vi "Link Read Parameters.vi"(7 "Parameter R Table in":refnum<class "Registry.lvclass">, 8 "error in (no error)":errorcluster, 11 "Major Frame in":refnum<class "Major Frame.lvclass">) -> (0 "error out":errorcluster, 5 "Parameter R Table out":refnum<class "Registry.lvclass">)   [LabVIEW 2020, in "BCI-1553 API.lvlib" / "Major Frame.lvclass"]
doc: "Links read-only transmit parameters to the Read Table."
uses:
  Major Frame.lvclass
  Dependencies/Registry/Registry.lvclass
  Major Frame.lvclass/Major Frame.ctl
  Dependencies/Registry/Registry.lvclass/Registry.ctl
  Message/Message.lvclass
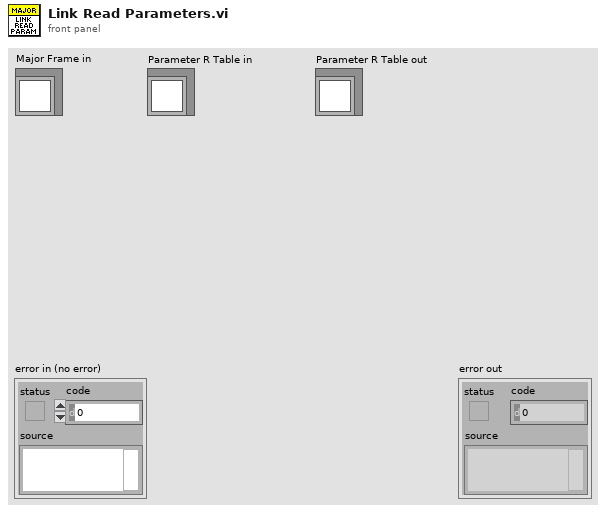
[diagram p1: front panel]
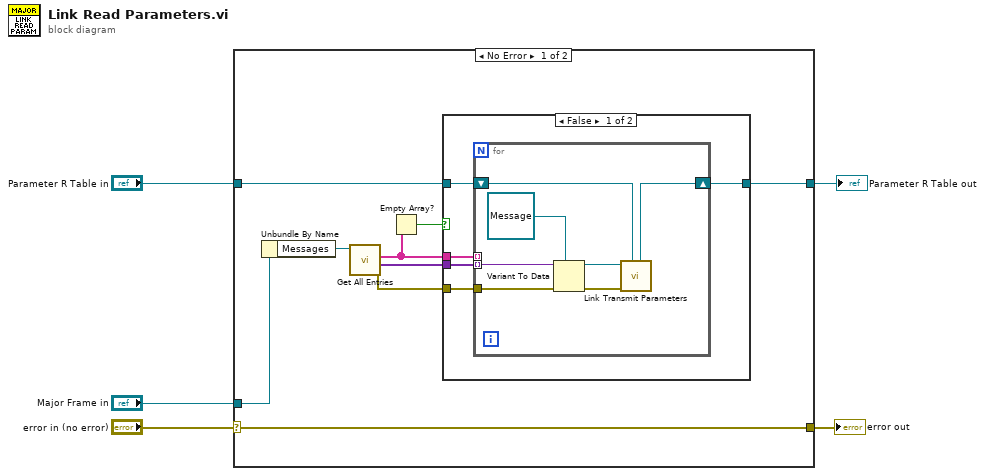
[diagram p0: block diagram]
diagram:
  n1 = case shown="No Error" "error in (no error)" {
    selector: "error in (no error)" -> [w14 w29]
    tunnel: [w14 w29] -> w4
    tunnel: "Major Frame in" -> [w13 _]
    tunnel: "Parameter R Table in" -> [w8 w28]
    tunnel: [w6 w28] -> w1
    frame No Error {
      n2 = Unbundle By Name(w13) -> ("Messages"=w12:refnum<class "Registry.lvclass">)
      n3 = call "Get All Entries.vi"("Registry in"=w12) -> ("error out"=w7:errorcluster, "Values"=w9:variant[], "Keys"=w10:string[])  [unwired: 8 in]
      n4 = Empty Array?(array=w10) -> (empty?=w11:bool)
      n5 = case shown="False" w11 {
        tunnel: w10 -> [w16 _]
        tunnel: w9 -> [w19 _]
        tunnel: w8 -> [w17 w27]
        tunnel: w7 -> [w18 _]
        tunnel: [w15 w27] -> w6
        frame False {
          n6 = for {
            tunnel: w19 -> [w26] mode=indexing
            tunnel: w18 -> [w25]
            shift-right: [w20] -> w15
            shift-left: w17 -> [w21]
            tunnel: w16 -> [_] mode=indexing
            n7 = Variant To Data(error in=w25, type=refnum<class "Message.lvclass"> refnum ("SLSC 1553 API.lvlib:Message.lvclass"), Variant=w26) -> (data=w23:refnum<class "Message.lvclass">, error out=w22:errorcluster)
            n8 = call "Link Transmit Parameters.vi"("Parameter R Table in"=w21, "error in (no error)"=w22, "Message in"=w23) -> ("Parameter R Table out"=w20:refnum<class "Registry.lvclass">)  [unwired: 7 in, 1 out]
          }
        }
        frame True {
        }
      }
    }
    frame Error {
    }
  }
  "error out" <- w4
  "Parameter R Table out" <- w1
